vi "Load cam video relative times from file.vi"(7 "Number of frames":i32, 9 "Acquisition time unknown":bool, 10 "Experiment Header's Statistics":T1, 11 "Binary file to read":path) -> (0 "Frame relative times array":i64[](array[numeric]), 1 "Elements to keep":bool[](array[boolean]), 2 "Frame numbers array":i64[](array[numeric]), 3 "Relative times file not found or error":bool)   [LabVIEW 2017]
uses:
  Typedefs/Test header stats cluster.ctl
panel:
  out "Number of valid frames":i32
  out "Relative times file path":path
  out "Number of original frames":i32
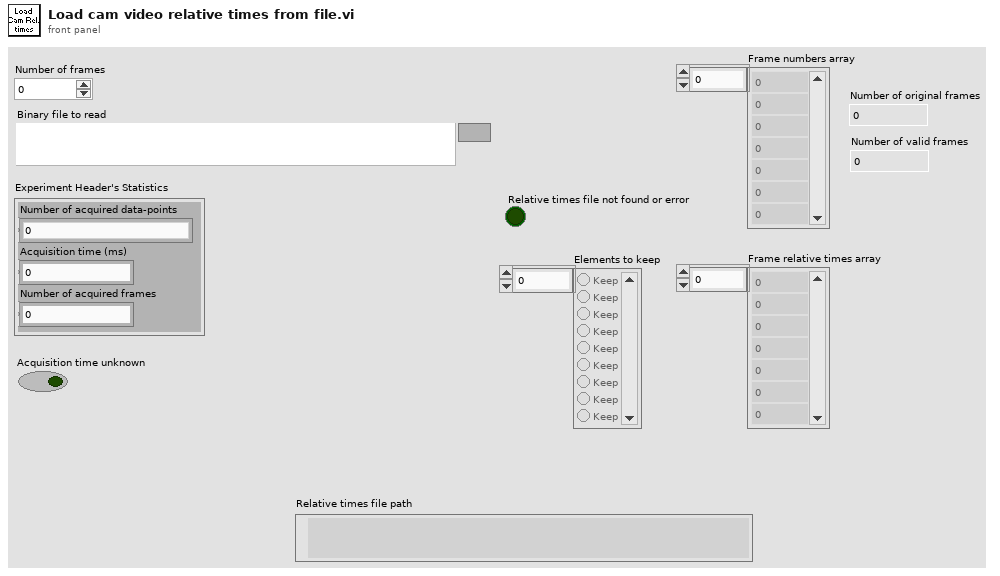
[diagram p1: front panel]
types:
  T1 = typedef "Test header stats cluster.ctl" = cluster{"Number of acquired data-points":dbl, "Acquisition time (ms)":dbl, "Number of acquired frames":dbl}
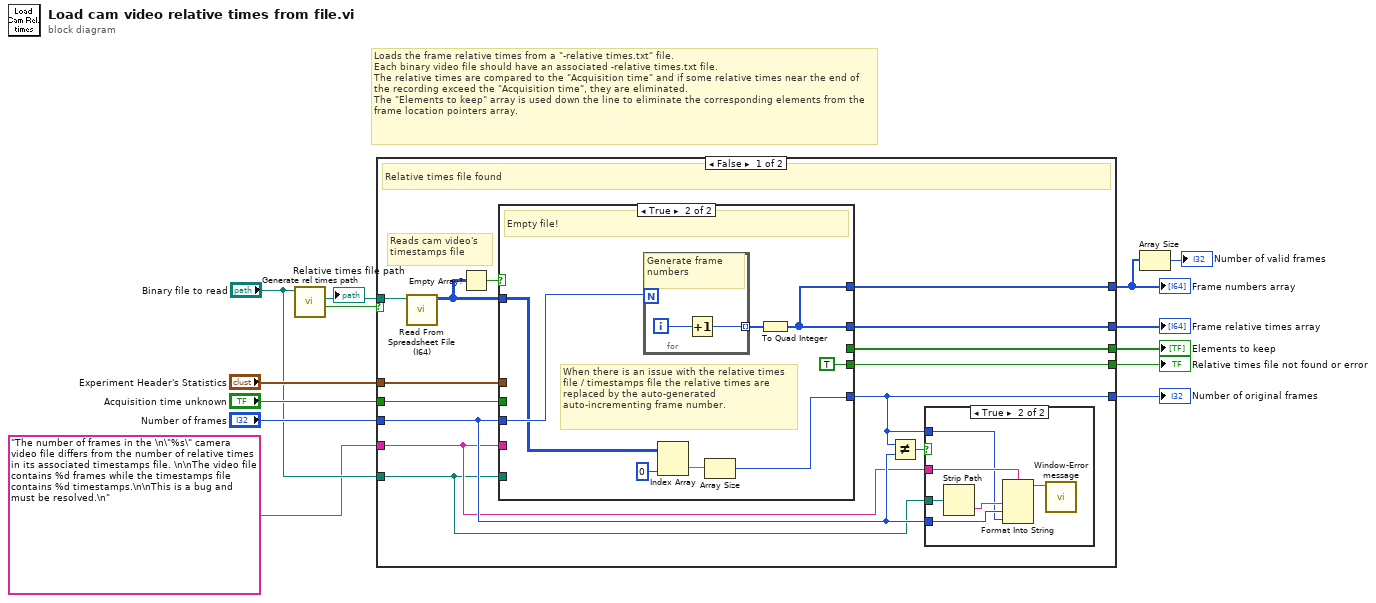
[diagram p0: block diagram]
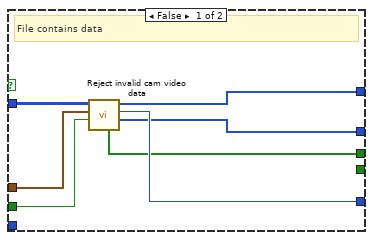
[diagram p3: hidden frame]
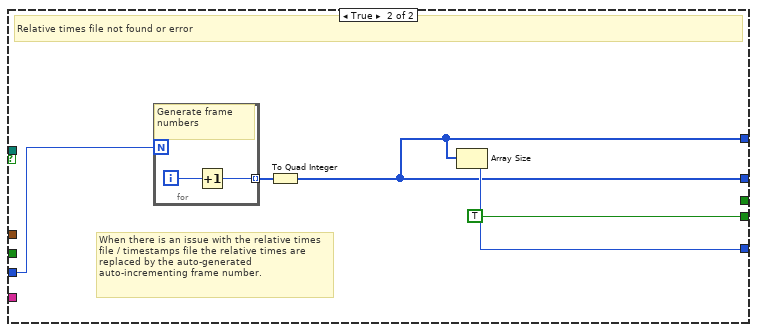
[diagram p4: hidden frame]
diagram:
  # "Loads the frame relative times from a \"-relative times.txt\" file.\nEach binary video file should have an associated -relative times.txt file.\nThe relative times are compared to the \"Acquisition time\" and if some relative times near the end of the recording exceed the \"Acquisition time\", they are eliminated.\nThe \"Elements to keep\" array is used down the line to eliminate the corresponding elements from the frame location pointers array."
  n1 = call "Generate rel times path.vi"("Binary file to read"="Binary file to read") -> ("Relative times file not found or error"=w13:bool, "Relative times file path"=w12:path)  [unwired: 9 in]
  "Relative times file path" <- w12
  n2 = case shown="False" w13 {
    tunnel: w12 -> [w21 _]
    tunnel: [w26 w51] -> w2
    tunnel: [w25 TRUE] -> w11
    tunnel: "Experiment Header's Statistics" -> [w24 _]
    tunnel: "Acquisition time unknown" -> [w23 _]
    tunnel: [w17 w52] -> w8
    tunnel: "Number of frames" -> [w16 w53]
    tunnel: [w22 _] -> w6
    tunnel: "The number of frames in the \n\"%s\" camera video file differs from the number of relative times in its associated timestamps file. \n\nThe video file contains %d frames while the timestamps file contains %d timestamps.\n\nThis is a bug and must be resolved.\n" ("Message") -> [w15 _]
    tunnel: "Binary file to read" -> [w14 _]
    tunnel: [w19 w51] -> w4
    frame False {
      # "Reads cam video's timestamps file"
      # "Relative times file found"
      n3 = call <vilib>:"Read From Spreadsheet File (I64).vi"("file path (dialog if empty)"=w21) -> ("all rows"=w20:i64[][])  [unwired: 6 in, 4 out]
      n4 = Empty Array?(array=w20) -> (empty?=w27:bool)
      n5 = case shown="False" w27 {
        tunnel: w20 -> [w40 w43]
        tunnel: [w35 w45] -> w26
        tunnel: [_ TRUE] -> w25
        tunnel: w24 -> [w39 _]
        tunnel: w23 -> [w38 _]
        tunnel: [w37 w41] -> w17
        tunnel: w16 -> [_ w46]
        tunnel: [w36 _] -> w22
        tunnel: w15 -> [_ _]
        tunnel: w14 -> [_ _]
        tunnel: [w34 w45] -> w19
        frame False {
          # "File contains data"
          n6 = call "Reject invalid cam video data.vi"("Acquisition time unknown"=w38, "Experiment Header's Statistics"=w39, "Cam video's timestamps file"=w40) -> ("Frame relative times array"=w34:i64[], "Number of original frames"=w37:i32, "Frame numbers array"=w35:i64[], "Elements to keep"=w36:bool[])  [unwired: 5 in]
        }
        frame True {
          # "When there is an issue with the relative times file / timestamps file the relative times are replaced by the auto-generated auto-incrementing frame number."
          # "Empty file!"
          n7 = for {
            N: w46 -> [_]
            tunnel: [w49] -> w47 mode=indexing
            i -> [w50]
            # "Generate frame numbers"
            n8 = Increment(x=w50) -> (x+1=w49:i32)
          }
          n9 = Index Array(array=w43, index (col)=0 ("disabled index (col)")) -> (element=w42:i64[])  [unwired: 1 in]
          n10 = Array Size(array=w42) -> (size(s)=w41:i32)
          n11 = To Quad Integer(1:w47) -> (0:w45:i64[])
        }
      }
      n12 = Not Equal?(x=w17, y=w16) -> (x != y?=w18:bool)
      n13 = case shown="True" w18 {
        tunnel: w15 -> [_ w33]
        tunnel: w14 -> [_ w32]
        tunnel: w16 -> [_ w30]
        tunnel: w17 -> [_ w28]
        frame False {
        }
        frame True {
          n14 = Strip Path(path=w32) -> (name=w31:string)  [unwired: 1 out]
          n15 = Format Into String(format string=w33, w31, w30, w28) -> (resulting string=w29:string)  [unwired: 2 in, 1 out]
          n16 = call "Window-Error message.vi"("Message"=w29) -> ()  [unwired: 10 in, 1 out]
        }
      }
    }
    frame True {
      # "When there is an issue with the relative times file / timestamps file the relative times are replaced by the auto-generated auto-incrementing frame number."
      # "Relative times file not found or error"
      n17 = for {
        N: w53 -> [_]
        tunnel: [w56] -> w54 mode=indexing
        i -> [w57]
        # "Generate frame numbers"
        n18 = Increment(x=w57) -> (x+1=w56:i32)
      }
      n19 = To Quad Integer(1:w54) -> (0:w51:i64[])
      n20 = Array Size(array=w51) -> (size(s)=w52:i32)
    }
  }
  "Frame numbers array" <- w2
  "Relative times file not found or error" <- w11
  "Number of original frames" <- w8
  "Elements to keep" <- w6
  "Frame relative times array" <- w4
  n21 = Array Size(array=w2) -> (size(s)=→"Number of valid frames":i32)
